vi "StartAllHomeMove.vi"(8 "error in (no error)":errorcluster, 9 "Positions to home":T1[](array[typedef])=[{"mmWave Axis"="BS1", "eng. value"=0.0}, {"mmWave Axis"="BS2", "eng. value"=0.0}, {"mmWave Axis"="RT1", "eng. value"=0.0}, {"mmWave Axis"="BS3", "eng. value"=0.0}, {"mmWave Axis"="BS4", "eng. value"=0.0}, {"mmWave Axis"="RT2", "eng. value"=0.0}, {"mmWave Axis"="RT3", "eng. value"=0.0}], 11 "VXMMotionManager in":refnum<class "VXMMotionManager.lvclass">) -> (0 "error out":errorcluster, 3 "VXMMotionManager out":refnum<class "VXMMotionManager.lvclass">)   [LabVIEW 2018, in "VXMMotionManager.lvclass"]
doc: "put home positions in the X,Y,Z,T target position and start moving."
uses:
  VXMMotionManager.lvclass
  APARMainSubvis/VXM Public API/singleAxisMoveDef.ctl
  APARMainSubvis/VXM Public API/mmWaveAxis.ctl
  MoveAllAbsoluteStates.ctl
  VXMMotionManager.lvclass/VXMMotionManager.ctl
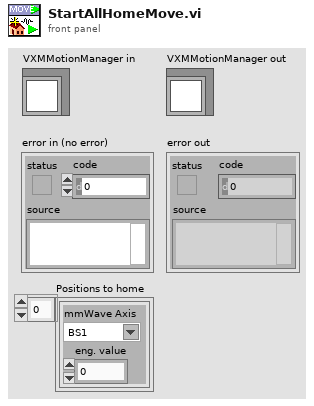
[diagram p1: front panel]
types:
  T1 = typedef "singleAxisMoveDef.ctl" = cluster{"mmWave Axis":T2, "eng. value":dbl}
  T2 = typedef "mmWaveAxis.ctl" = string
  T3 = typedef "VXMMotionManager.lvclass/MoveAllAbsoluteStates.ctl" = enum16{"start next move", "wait motion end"}
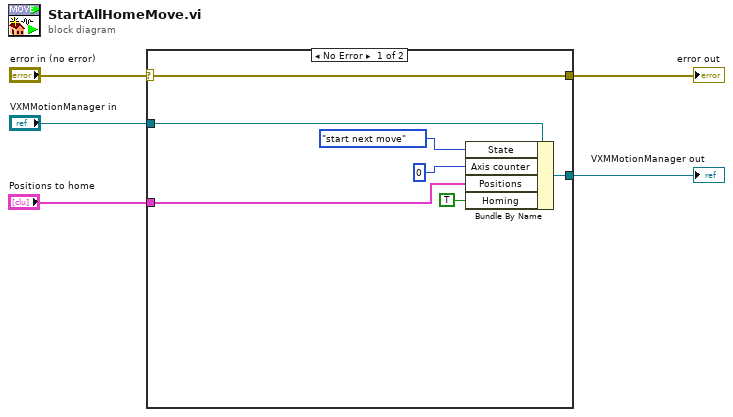
[diagram p0: block diagram]
diagram:
  n1 = case shown="No Error" "error in (no error)" {
    selector: "error in (no error)" -> [w12 w14]
    tunnel: [w12 w14] -> w4
    tunnel: [w8 w13] -> w3
    tunnel: "VXMMotionManager in" -> [w7 w13]
    tunnel: "Positions to home" -> [w6 _]
    frame No Error {
      n2 = Bundle By Name(cluster=w7, "State"=MoveAllAbsoluteStates."start next move", "Axis counter"=0 ("Axis (0-3)"), "Positions"=w6, "Homing"=TRUE) -> (w8:refnum<class "VXMMotionManager.lvclass">)
    }
    frame Error {
    }
  }
  "error out" <- w4
  "VXMMotionManager out" <- w3
